vi "SystKeyDecoder.vi"(1 "1D array":bool[](array[boolean])) -> (0 "String":string)   [LabVIEW 2017]
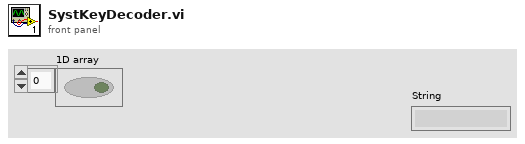
[diagram p1: front panel]
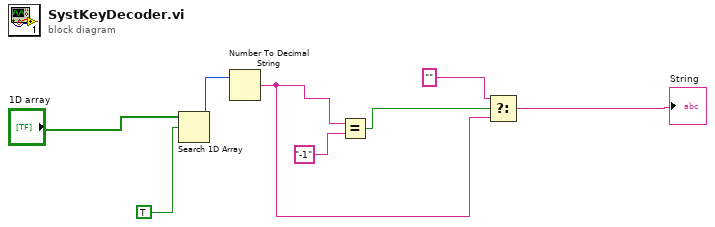
[diagram p0: block diagram]
diagram:
  n1 = Search 1D Array(1D array="1D array", element=TRUE) -> (index of element=w8:i32)  [unwired: 1 in]
  n2 = Number To Decimal String(number=w8) -> (decimal integer string=w4:string)  [unwired: 1 in]
  n3 = Equal?(x=w4, y="-1") -> (x = y?=w6:bool)
  n4 = Select(t="" ("f"), s=w6, f=w4) -> (s? t:f=→"String":string)
